vi "Finalize.vi"(8 "error in (no error)":errorcluster, 11 "ConfirmQuitSpecPage in":refnum<class "ConfirmQuitSpecPage.lvclass">) -> (0 "error out":errorcluster, 2 "MetaDataObj out":refnum<class "MetaDataObj.lvclass">, 3 "ConfirmQuitSpecPage out":refnum<class "ConfirmQuitSpecPage.lvclass">)   [LabVIEW 2016, in "ConfirmQuitSpecPage.lvclass"]
uses:
  <resource>/dialog/NewProjectWizard/SpecPage/ConfirmQuitSpecPage/ConfirmQuitSpecPage.lvclass
  <resource>/dialog/NewProjectWizard/MetaDataObj/MetaDataObj.lvclass
  <resource>/dialog/NewProjectWizard/SpecPage/ConfirmQuitSpecPage/ConfirmQuitSpecPage.lvclass/ConfirmQuitSpecPage.ctl
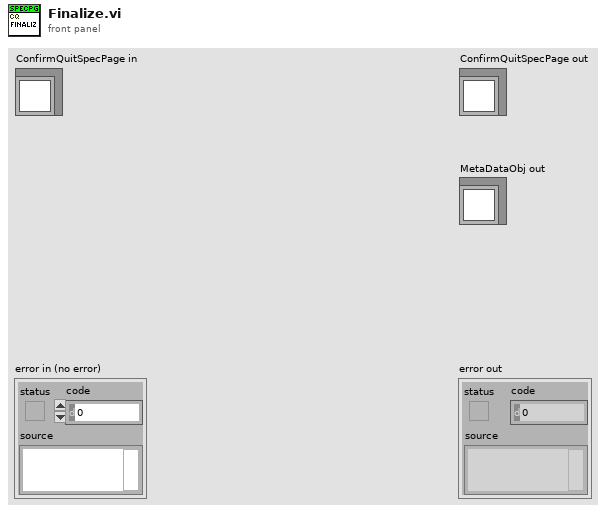
[diagram p1: front panel]
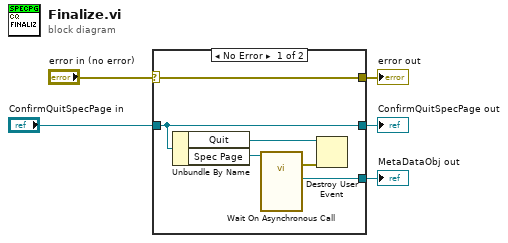
[diagram p0: block diagram]
diagram:
  n1 = case shown="No Error" "error in (no error)" {
    selector: "error in (no error)" -> [w6 w13]
    tunnel: [w6 w13] -> w4
    tunnel: [w11 w12] -> w2
    tunnel: "ConfirmQuitSpecPage in" -> [w11 w12]
    tunnel: [w8 _] -> w1
    frame No Error {
      n2 = Unbundle By Name(w11) -> ("Quit"=w10:refnum<user-event>, "Spec Page"=w9:refnum<vi>)
      n3 = call-by-ref "Wait On Asynchronous Call"(reference=w9) -> (error out=w7:errorcluster, "MetaDataObj out"=w8:refnum<class "MetaDataObj.lvclass">)  [unwired: 12 in, 1 out]
      n4 = Destroy User Event(user event=w10, error in=w7) -> ()  [unwired: 1 out]
    }
    frame Error {
    }
  }
  "error out" <- w4
  "ConfirmQuitSpecPage out" <- w2
  "MetaDataObj out" <- w1
